vi "get_max_peaks.vi"() -> ()   [LabVIEW 2020]
panel:
  out "end state":string
  in  "crossings":dbl[](array[numeric])
  in  "times":dbl[](array[numeric])
  in  "p->n indexes":i32[](array[numeric])
  in  "n->p indexes":i32[](array[numeric])
  in  "p->n crossing?":bool[](array[boolean])
  in  "n->p crossing?":bool[](array[boolean])
  in  "locations (interpolated indexes)":dbl[](array[numeric])
  in  "amplitudes":dbl[](array[numeric])
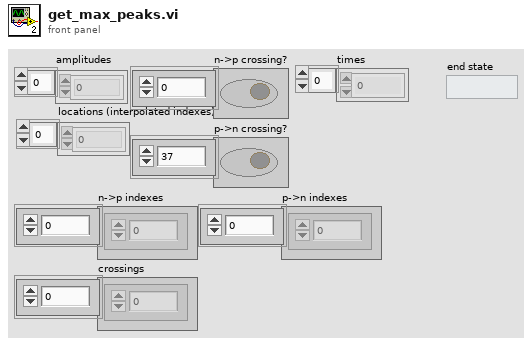
[diagram p1: front panel]
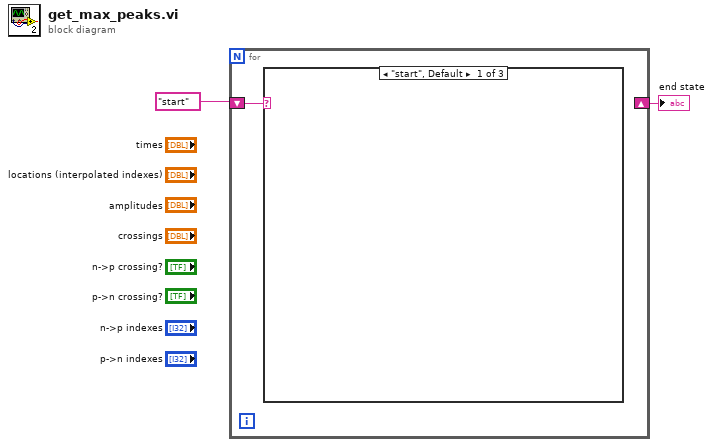
[diagram p0: block diagram]
diagram:
  n1 = for {
    shift-right: [_] -> w1
    shift-left: "start" ("Combo Box") -> [w3]
    n2 = case shown="\"start\", Default" w3 {
      frame "start", Default {
      }
      frame "get peaks" {
      }
      frame "evaluate" {
      }
    }
  }
  "end state" <- w1
